vi "Save ID Behind Path.vi"(8 "Error In":errorcluster, 9 "Paths":string, 10 "IDs":string, 11 "Paths Dict":variant) -> (0 "Error Out":errorcluster, 3 "Paths Dict":variant)   [LabVIEW 2020, in "NI_VIAnCFGDataStructure.lvlib" / "Tree.lvclass"]
uses:
  <vilib>/addons/analyzer/VIAnCFGDataStructure/Tree Manager/Tree.lvclass
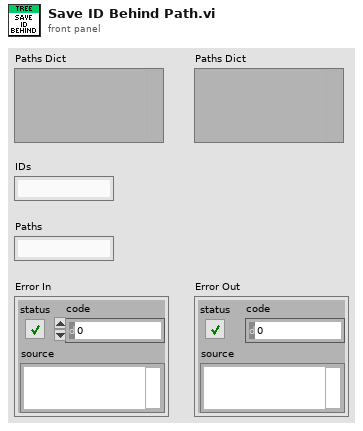
[diagram p1: front panel]
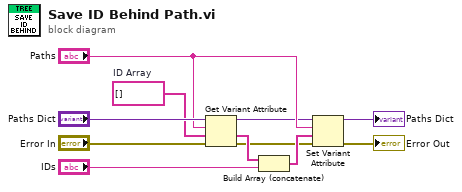
[diagram p0: block diagram]
diagram:
  w5 = string[] []  # ID Array
  n1 = Get Variant Attribute(Variant="Paths Dict", name="Paths", default value (empty Variant)=w5, error in="Error In") -> (duplicate Variant=w4:variant, value=w3:string[], error out=w1:errorcluster)  [unwired: 1 out]
  n2 = Build Array (concatenate)(w3, "IDs") -> (w2:string[])
  n3 = Set Variant Attribute(Variant=w4, name="Paths", value=w2, error in=w1) -> (Variant out=→"Paths Dict":variant, error out=→"Error Out":errorcluster)  [unwired: 1 out]
